vi "Line Detector Read File.vi"(8 "error in (no error)":errorcluster, 10 "File":path=path "C:/Data/April_2017/042017/ru112_042017.tdms", 11 "Line Detector Configuration":T2={"Peak width guess"=500.0, "Background removal"=enum."High-pass", "Smoothing"=enum."Low-pass", "Smooth window"=200.0, "Relative threshold"=0.2, "Finder algorithm"=enum."Wavelet", "Bgd window"=50000.0, "Spectrum recorder module name"="Spectrum Recorder", "Fit window"=1000.0, "Initial fit guess"=enum."Peak finder", "Follow\npeaks"=FALSE, "Re-sample"=nan, "Tolerance"=1000.0, "Max iterations"=1000} {"Tolerance" format="%#_6e"; "Re-sample" format="%#_6pHz"; "Fit window" format="%#_6pHz"; "Bgd window" format="%#_6pHz"; "Smooth window" format="%#_6pHz"; "Peak width guess" format="%#_6pHz"}) -> (0 "error out":errorcluster, 1 "Internal Spectrum Configuration":T1={"Start frequency"=500000.0, "End frequency"=2000000.0, "Coarse step"=100.0, "Step duration"=0.004, "Red Pitaya address"="192.168.1.100", "Open plot \non start"=FALSE, "Fine region centers"=[], "Regions width"=1.0, "Fine step"=0.0, "Pause between scans"=0.0, "Clear rgs on start"=FALSE, "Output amplitude"=1.0} {"Output amplitude" min=0.0 max=1.0 step=0.1 format="%#_6pV"; "Pause between scans" format="%#_6ps"; "Fine step" min=0.001 format="%#_6pHz"; "Regions width" format="%#_6pHz"; "Fine region centers" format="%#_6pHz"; "Step duration" format="%#_6ps"; "Coarse step" format="%#_6pHz"; "End frequency" format="%#_6pHz"; "Start frequency" format="%#_6pHz"}, 2 "File out":path, 3 "Signal Y":dbl[](array[numeric]), 4 "found?":bool, 5 "Signal X":dbl[](array[numeric]), 6 "sp time":timestamp, 7 "Frequency":dbl[](array[numeric]), 9 "Fine region centers":dbl[](array[numeric]))   [LabVIEW 2020]
uses:
  LabActor/Post-Processors/Line Detector/Resonance Detector Configuration.ctl
  Red Pitaya/RP Core/Red Pitaya Transceiver Driver/Internal Spectrum Configuration.ctl
panel:
  out "dt":dbl
  # "Peak finder config"
  # "Lorentzian fit config"
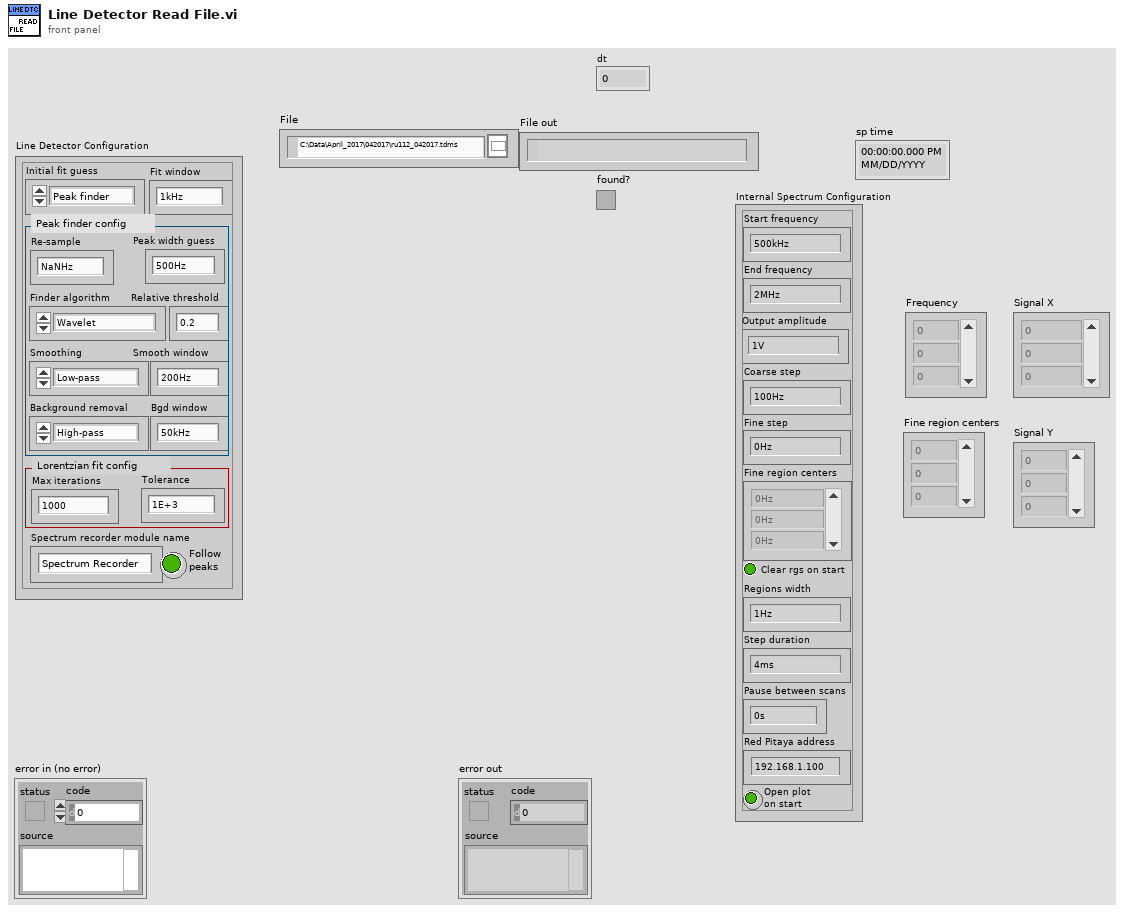
[diagram p1: front panel]
types:
  T1 = typedef "Internal Spectrum Configuration.ctl" = cluster{"Start frequency":dbl, "End frequency":dbl, "Coarse step":dbl, "Step duration":dbl, "Red Pitaya address":string, "Open plot \non start":bool, "Fine region centers":dbl[], "Regions width":dbl, "Fine step":dbl, "Pause between scans":dbl, "Clear rgs on start":bool, "Output amplitude":dbl}
  T2 = typedef "Resonance Detector Configuration.ctl" = cluster{"Peak width guess":dbl, "Background removal":enum16{"NONE", "High-pass", "Detrend"}, "Smoothing":enum16{"NONE", "Low-pass", "Denoise"}, "Smooth window":dbl, "Relative threshold":dbl, "Finder algorithm":enum16{"Basic", "Wavelet", "Wavelet+detrend"}, "Bgd window":dbl, "Spectrum recorder module name":string, "Fit window":dbl, "Initial fit guess":enum16{"Peak finder", "Last fit"}, "Follow\npeaks":bool, "Re-sample":dbl, "Tolerance":dbl, "Max iterations":i32}
  T3 = enum16{"open", "open or create", "create or replace", "create", "open (read-only)"}
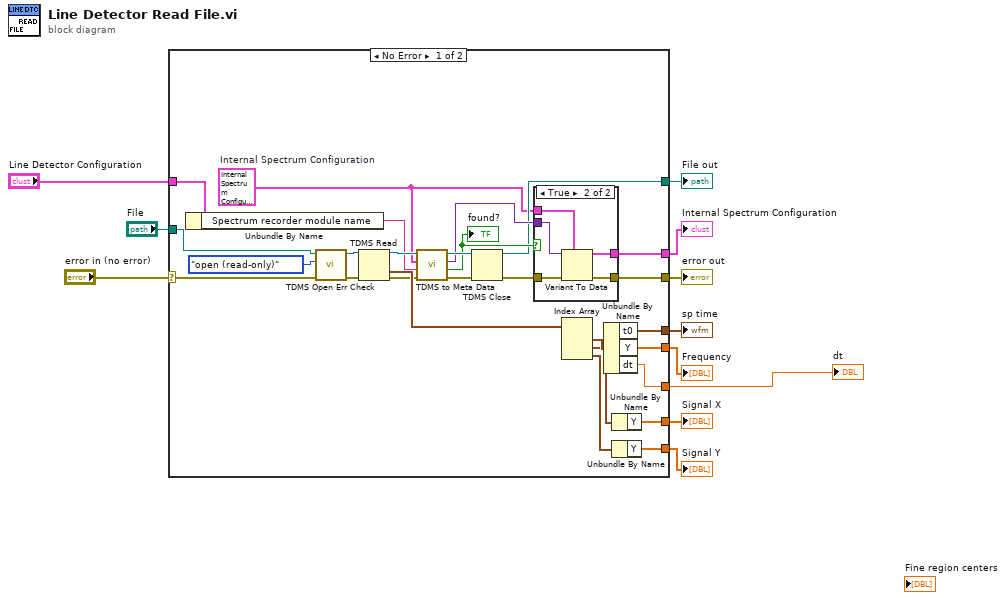
[diagram p0: block diagram]
diagram:
  n1 = case shown="No Error" "error in (no error)" {
    selector: "error in (no error)" -> [w30 w45]
    tunnel: "File" -> [w31 w46]
    tunnel: [w19 w46] -> w9
    tunnel: "Line Detector Configuration" -> [w14 _]
    tunnel: [w21 w45] -> w7
    tunnel: [w29 _] -> w6
    tunnel: [w20 _] -> w5
    tunnel: [w18 _] -> w4
    tunnel: [w17 _] -> w3
    tunnel: [w16 _] -> w2
    tunnel: [w12 _] -> w1
    frame No Error {
      w15 = T1 {"Start frequency"=500000.0, "End frequency"=2000000.0, "Coarse step"=40.0, "Step duration"=0.004, "Red Pitaya address"="192.168.1.100", "Open plot \non start"=FALSE, "Fine region centers"=[], "Regions width"=1.0, "Fine step"=0.0, "Pause between scans"=0.0, "Clear rgs on start"=FALSE, "Output amplitude"=1.0}  # Internal Spectrum Configuration
      n2 = Unbundle By Name(w14) -> ("Spectrum recorder module name"=w13:string)
      n3 = call "TDMS Open Err Check.vi"("Error In"=w30, "operation (0:open)"=T3."open (read-only)", "File Path Control"=w31) -> ("Error Out"=w36:errorcluster, "tdms file out"=w37:refnum<k34>)  [unwired: 6 in, 1 out]
      n4 = TDMS Read(0:w37, 11:w36) -> (4:w28:refnum<k34>, 10:w35:waveform(dbl)[], 15:w27:errorcluster)  [unwired: 6 in, 3 out]
      n5 = call "TDMS to Meta Data.vi"("Error In"=w27, "Name"=w13, "Value"=w15, "tdms file"=w28) -> ("Error Out"=w26:errorcluster, "found?"=w24:bool, "Variant out"=w22:variant, "tdms file out"=w25:refnum<k34>)  [unwired: 4 in]
      "found?" <- w24
      n6 = TDMS Close(8:w26, 11:w25) -> (0:w23:errorcluster, 3:w19:path)
      n7 = case shown="True" w24 {
        tunnel: w23 -> [w39 w44]
        tunnel: w15 -> [_ w43]
        tunnel: w22 -> [_ w42]
        tunnel: [w39 w41] -> w21
        tunnel: [_ w40] -> w20
        frame False {
        }
        frame True {
          n8 = Variant To Data(error in=w44, type=w43, Variant=w42) -> (data=w40:T1, error out=w41:errorcluster)
        }
      }
      n9 = Index Array(array=w35) -> (element #1=w34:waveform(dbl), element #2=w32:waveform(dbl), element #3=w33:waveform(dbl))  [unwired: 3 in]
      n10 = Unbundle By Name(w34) -> ("t0"=w29:timestamp, "Y"=w18:dbl[], "dt"=w12:dbl)
      n11 = Unbundle By Name(w32) -> ("Y"=w17:dbl[])
      n12 = Unbundle By Name(w33) -> ("Y"=w16:dbl[])
    }
    frame Error {
    }
  }
  "error out" <- w7
  "File out" <- w9
  "sp time" <- w6
  "Internal Spectrum Configuration" <- w5
  "Frequency" <- w4
  "Signal X" <- w3
  "Signal Y" <- w2
  "dt" <- w1
